vi "_Step Counter.Step Count Controller - FG.vi"(0 "Step Action":T1=enum."Get Step") -> (6 "Step":string)   [LabVIEW 2018]
uses:
  Step Counter.Action.ctl
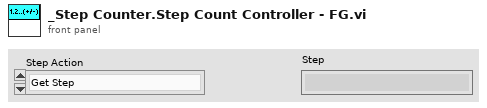
[diagram p1: front panel]
types:
  T1 = typedef "Step Counter.Action.ctl" = enum16{"Init", "Section Start", "Data +", "Sub Section Start", "Sub Section End", "Get Step"}
  T2 = typedef "Step Counter.Action.ctl" = enum16{"Init", "Inc +", "Level Up <-", "Top Level  +", "Level Dwn ->", "Get Step"}
  T3 = cluster{"Level":i32, "Cnts":i32[], "Step":string}
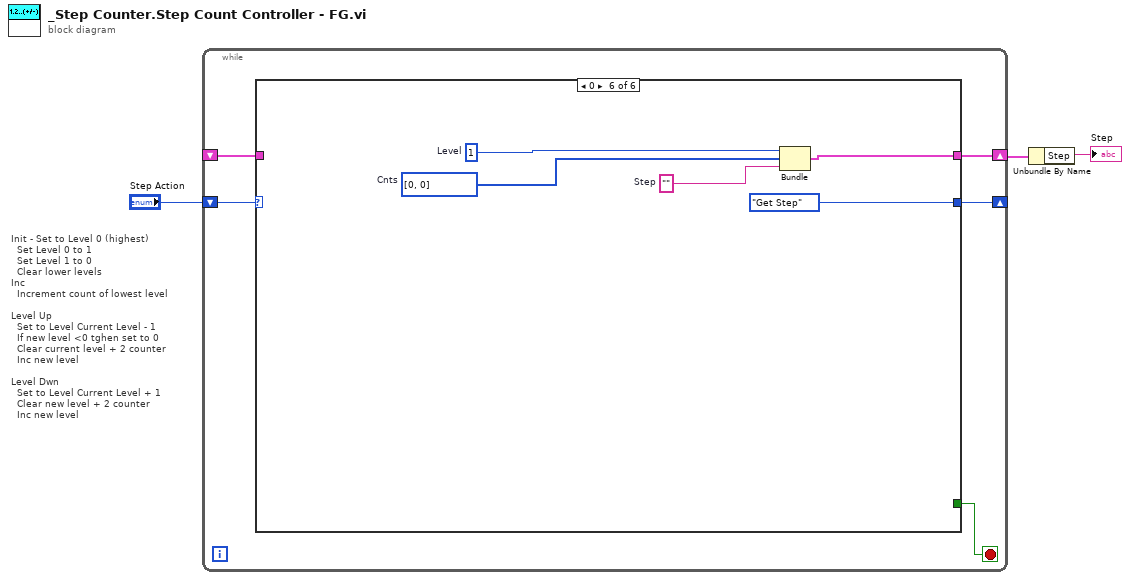
[diagram p0: block diagram]
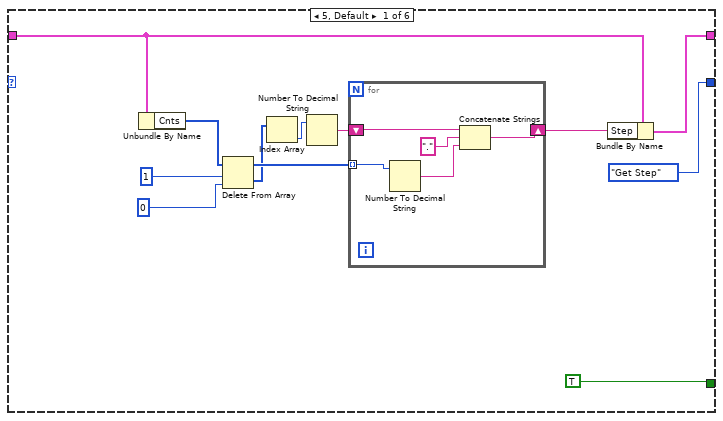
[diagram p2: hidden frame]
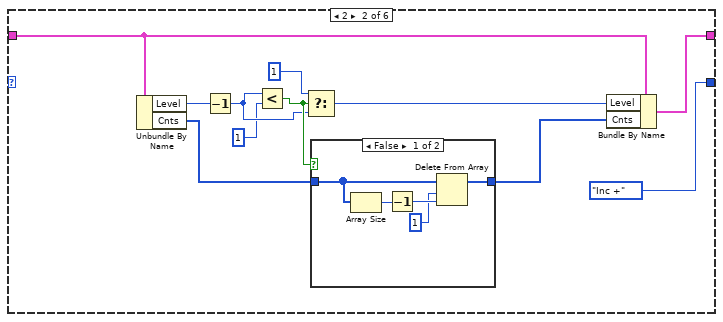
[diagram p3: hidden frame]
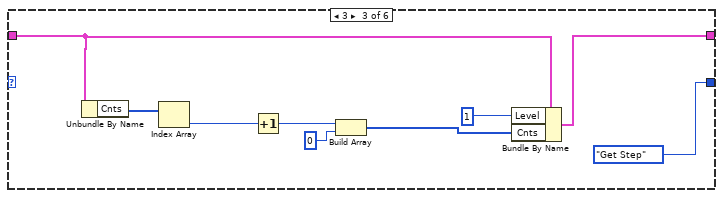
[diagram p5: hidden frame]
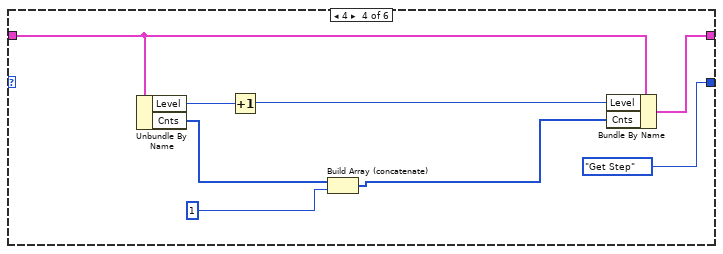
[diagram p6: hidden frame]
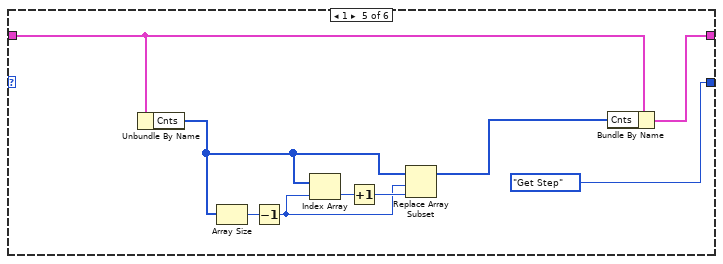
[diagram p7: hidden frame]
diagram:
  # "Init - Set to Level 0 (highest)\n  Set Level 0 to 1\n  Set Level 1 to 0\n  Clear lower levels\nInc\n  Increment count of lowest level\n\nLevel Up\n  Set to Level Current Level - 1\n  If new level <0 tghen set to 0\n  Clear current level + 2 counter\n  Inc new level\n\nLevel Dwn\n  Set to Level Current Level + 1\n  Clear new level + 2 counter\n  Inc new level"
  n1 = while {
    shift-right: [w8] -> w2
    shift-left: _ -> [w7]
    shift-right: [w4] -> _
    shift-left: "Step Action" -> [w6]
    stop <- w5 stop-if-true
    n2 = case shown="0" w6 {
      tunnel: [w15 w35 w50 w58 w67 w71] -> w8
      tunnel: w7 -> [w16 w36 w49 w59 w68 _]
      tunnel: [TRUE _ _ _ _ _] -> w5
      tunnel: [Step_Counter.Action."Get Step" ("Step Action") Step_Counter.Action."Inc +" ("Step Action") Step_Counter.Action."Get Step" ("Step Action") Step_Counter.Action."Get Step" ("Step Action") Step_Counter.Action."Get Step" ("Step Action") Step_Counter.Action."Get Step" ("Step Action")] -> w4
      frame 5, Default {
        n3 = Unbundle By Name(w16) -> ("Cnts"=w19:i32[])
        n4 = Delete From Array(array=w19, length=1, index=0) -> (deleted portion=w10:i32[], array with subset deleted=w18:i32[])
        n5 = Index Array(array=w10) -> (element=w11:i32)  [unwired: 1 in]
        n6 = Number To Decimal String(number=w11) -> (decimal integer string=w17:string)  [unwired: 1 in]
        n7 = for {
          tunnel: w18 -> [w23] mode=indexing
          shift-right: [w24] -> w14
          shift-left: w17 -> [w25]
          n8 = Number To Decimal String(number=w23) -> (decimal integer string=w22:string)  [unwired: 1 in]
          n9 = Concatenate Strings(w25, ".", w22) -> (w24:string)
        }
        n10 = Bundle By Name(cluster=w16, "Step"=w14) -> (w15:T3)
      }
      frame 2 {
        n11 = Unbundle By Name(w36) -> ("Level"=w34:i32, "Cnts"=w32:i32[])
        n12 = Decrement(x=w34) -> (x-1=w27:i32)
        n13 = Less?(x=w27, y=1) -> (x < y?=w28:bool)
        n14 = Select(t=1, s=w28, f=w27) -> (s? t:f=w31:i32)
        n15 = case shown="False" w28 {
          tunnel: w32 -> [w41 w42]
          tunnel: [w37 w42] -> w30
          frame False {
            n16 = Array Size(array=w41) -> (size(s)=w40:i32)
            n17 = Decrement(x=w40) -> (x-1=w39:i32)
            n18 = Delete From Array(array=w41, length=1, index=w39) -> (array with subset deleted=w37:i32[])  [unwired: 1 out]
          }
          frame True {
          }
        }
        n19 = Bundle By Name(cluster=w36, "Level"=w31, "Cnts"=w30) -> (w35:T3)
      }
      frame 3 {
        n20 = Unbundle By Name(w49) -> ("Cnts"=w48:i32[])
        n21 = Index Array(array=w48) -> (element=w47:i32)  [unwired: 1 in]
        n22 = Increment(x=w47) -> (x+1=w46:i32)
        n23 = Build Array(w46, 0 ("element")) -> (w43:i32[])
        n24 = Bundle By Name(cluster=w49, "Level"=1 ("element"), "Cnts"=w43) -> (w50:T3)
      }
      frame 4 {
        n25 = Unbundle By Name(w59) -> ("Level"=w57:i32, "Cnts"=w56:i32[])
        n26 = Increment(x=w57) -> (x+1=w53:i32)
        n27 = Build Array (concatenate)(w56, 1) -> (w54:i32[])
        n28 = Bundle By Name(cluster=w59, "Level"=w53, "Cnts"=w54) -> (w58:T3)
      }
      frame 1 {
        n29 = Unbundle By Name(w68) -> ("Cnts"=w63:i32[])
        n30 = Array Size(array=w63) -> (size(s)=w66:i32)
        n31 = Decrement(x=w66) -> (x-1=w62:i32)
        n32 = Index Array(array=w63, index=w62) -> (element=w65:i32)
        n33 = Increment(x=w65) -> (x+1=w64:i32)
        n34 = Replace Array Subset(array=w63, new element=w64, index=w62) -> (w61:i32[])
        n35 = Bundle By Name(cluster=w68, "Cnts"=w61) -> (w67:T3)
      }
      frame 0 {
        w70 = ""  # Step
        w72 = i32[] [0, 0]  # Cnts
        w73 = 1  # Level
        n36 = Bundle("Level"=w73, "Cnts"=w72, "Step"=w70) -> (w71:T3)  [unwired: 1 in]
      }
    }
  }
  n37 = Unbundle By Name(w2) -> ("Step"=→"Step":string)
